vi "gen_drive_waveform_ramp_only.vi"(9 "ramping cycles":dbl, 11 "no of cycles":dbl=6000.0) -> (0 "signal out":waveform(dbl))   [LabVIEW 2019]
uses:
  <vilib>/Analysis/1siggen.llb/Ramp Pattern by Samples.vi
  global_variables.vi
  <vilib>/measure/NI_MABase.lvlib
  <vilib>/Analysis/NI_AALBase.lvlib
panel:
  out "Ramped output waveform":dbl[](graph)
  out "Original output waveform":dbl[](graph)
  out "Ramp Pattern":dbl[](graph)
  out "sample rate (from global)":dbl=500000.0 format="%#_6p"
  out "Transmit amplitude (from global)":dbl=3.3
  out "Transmit frequency (from global)":dbl=25000.0 format="%#_6p"
  out "Sample points per cycle":dbl
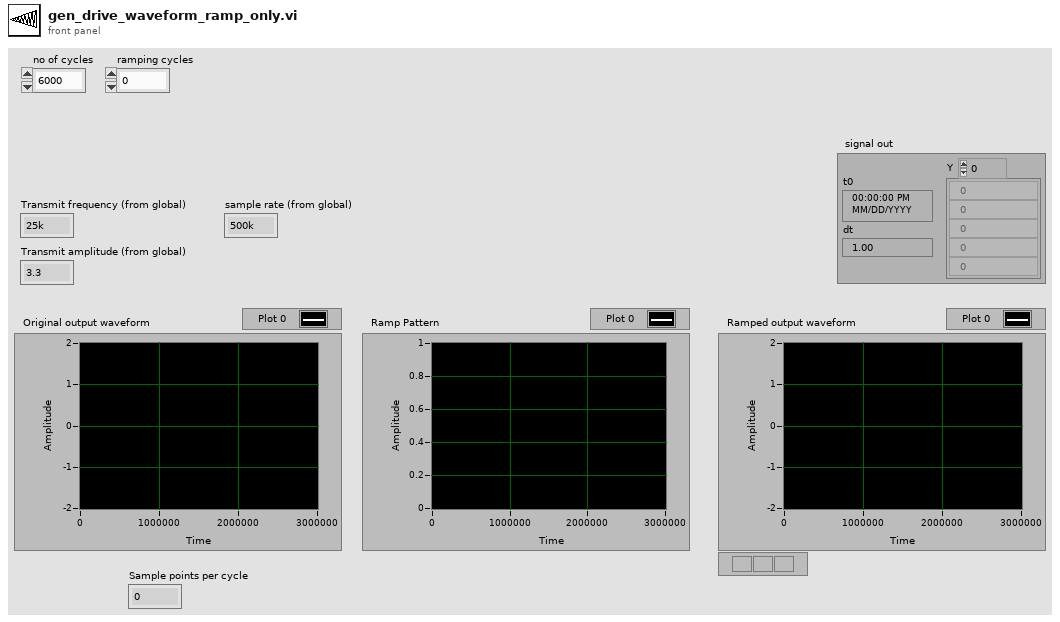
[diagram p1: front panel]
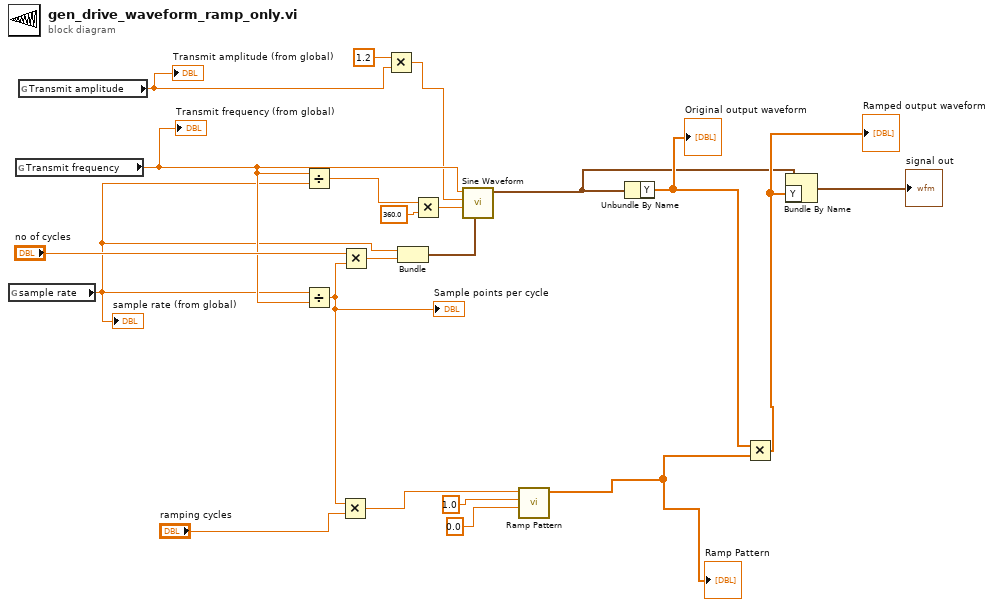
[diagram p0: block diagram]
diagram:
  n1 = global read "global_variables.vi" "sample rate"() -> (w15:dbl)
  "sample rate (from global)" <- w15
  n2 = global read "global_variables.vi" "Transmit frequency"() -> (w16:dbl)
  "Transmit frequency (from global)" <- w16
  n3 = global read "global_variables.vi" "Transmit amplitude"() -> (w2:dbl)
  "Transmit amplitude (from global)" <- w2
  n4 = Divide(x=w16, y=w15) -> (x/y=w20:dbl)
  n5 = Divide(x=w15, y=w16) -> (x/y=w12:dbl)
  "Sample points per cycle" <- w12
  n6 = Multiply(x=w12, y="ramping cycles") -> (x*y=w10:dbl)
  n7 = Multiply(x="no of cycles", y=w12) -> (x*y=w11:dbl)
  n8 = Multiply(x=1.2, y=w2) -> (x*y=w1:dbl)
  n9 = Bundle("sample rate"=w15, w11) -> (w21:cluster{"sample rate":dbl, dbl})  [unwired: 1 in]
  n10 = Multiply(x=w20, y=360.0) -> (x*y=w18:dbl)
  n11 = call <vilib>:"Sine Waveform.vi"("sampling info"=w21, "phase"=w18, "amplitude"=w1, "frequency"=w16) -> ("signal out"=w7:waveform(dbl))  [unwired: 6 in, 1 out]
  n12 = call-poly <vilib>:"Ramp Pattern.vi"("start"=0.0, "end"=1.0, "samples"=w10) -> ("Ramp Pattern"=w4:dbl[])  [unwired: 7 in, 1 out]
  "Ramp Pattern" <- w4
  n13 = Unbundle By Name(w7) -> ("Y"=w9:dbl[])
  "Original output waveform" <- w9
  n14 = Multiply(x=w9, y=w4) -> (x*y=w8:dbl[])
  "Ramped output waveform" <- w8
  n15 = Bundle By Name(cluster=w7, "Y"=w8) -> (→"signal out":waveform(dbl))
